vi "Init-Window.vi"(8 "error in (no error)":errorcluster, 11 "GLF Window in":refnum<class "Window.lvclass">) -> (0 "error out":errorcluster, 3 "GLF Window out":refnum<class "Window.lvclass">)   [LabVIEW 2020, in "GLF.lvlib" / "Window.lvclass"]
uses:
  Window.lvclass
  Window.lvclass/Window.ctl
  Engine/Engine.lvclass
  IAmGLF/IAmGLF.lvclass
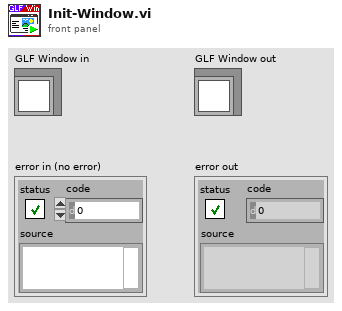
[diagram p1: front panel]
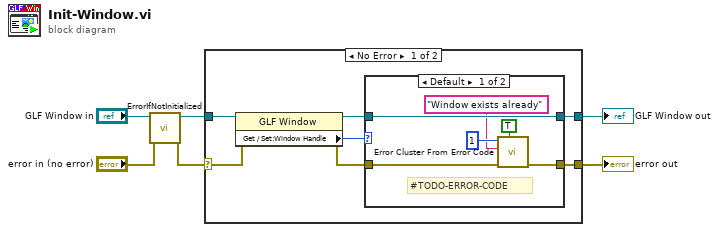
[diagram p0: block diagram]
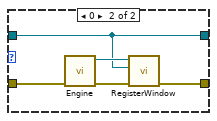
[diagram p2: hidden frame]
diagram:
  n1 = call "ErrorIfNotInitialized.vi"("error in (no error)"="error in (no error)", "IAmGLF in"="GLF Window in") -> ("error out"=w1:errorcluster, "IAmGLF out"=w3:refnum<class "Window.lvclass">)  [unwired: 8 in]
  n2 = case shown="No Error" w1 {
    selector: w1 -> [w11 w25]
    tunnel: [w13 w25] -> w6
    tunnel: w3 -> [w12 w26]
    tunnel: [w7 w26] -> w5
    frame No Error {
      n3 = property class="GLF Window"(reference=w12, error in=w11) -> (reference out=w8:refnum<class "Window.lvclass">, error out=w10:errorcluster, "Get / Set:Window Handle"=w9:i64)
      n4 = case shown="Default" w9 {
        tunnel: [w17 w22] -> w13
        tunnel: w8 -> [w19 w20]
        tunnel: w10 -> [w18 w21]
        tunnel: [w19 w20] -> w7
        frame Default {
          # "#TODO-ERROR-CODE"
          n5 = call <vilib>:"Error Cluster From Error Code.vi"("show call chain? (False)"=TRUE, "error in (no error)"=w18, "error message (\"\")"="Window exists already" ("error message (\"\")"), "error code (0)"=1) -> ("error out"=w17:errorcluster)  [unwired: 5 in]
        }
        frame 0 {
          n6 = call "Engine.vi"("error in (no error)"=w21) -> ("error out"=w23:errorcluster, "Engine"=w24:refnum<class "Engine.lvclass">)  [unwired: 9 in]
          n7 = call "RegisterWindow.vi"("error in (no error)"=w23, "Window"=w20, "Engine in"=w24) -> ("error out"=w22:errorcluster)  [unwired: 7 in, 1 out]
        }
      }
    }
    frame Error {
    }
  }
  "error out" <- w6
  "GLF Window out" <- w5
